vi "Matches.vi"(8 "error in (no error)":errorcluster, 10 "Actual":variant, 11 "Collection Contains in":refnum<class "Collection Contains.lvclass">) -> (0 "error out":errorcluster, 2 "Result":bool, 3 "Collection Contains out":refnum<class "Collection Contains.lvclass">)   [LabVIEW 2017, in "Transparent Assertions.lvlib" / "Collection Contains.lvclass"]
doc: "Evaluates the constraint for <B>Actual</B>. Returns true if the constraint is met."
uses:
  Collection Contains.lvclass
  Collection Contains.lvclass/Collection Contains.ctl
  Transparent Assertions.lvlib
  <vilib>/Utility/Data Type/NI_Data Type.lvlib
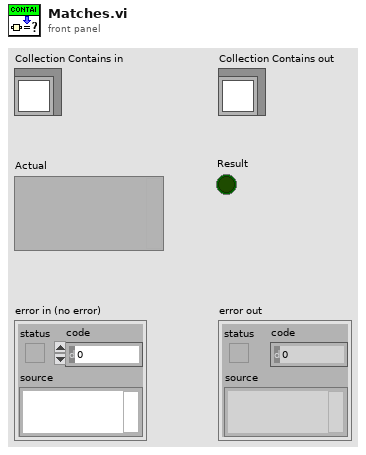
[diagram p1: front panel]
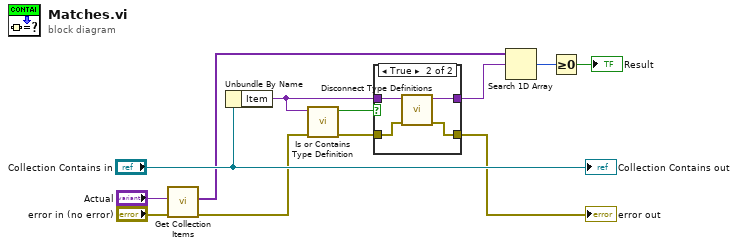
[diagram p0: block diagram]
diagram:
  n1 = call "Get Collection Items.vi"("error in (no error)"="error in (no error)", "Collection"="Actual") -> ("error out"=w3:errorcluster, "Items"=w8:variant[])  [unwired: 8 in]
  n2 = Unbundle By Name("Collection Contains in") -> ("Item"=w4:variant)
  n3 = call <vilib>:"Is or Contains Type Definition.vi"("error in (no error)"=w3, "Variant"=w4) -> ("error out"=w2:errorcluster, "Is or Contains Typedef"=w1:bool)  [unwired: 8 in]
  n4 = case shown="True" w1 {
    tunnel: [w13 w18] -> w6
    tunnel: [w14 w17] -> w5
    tunnel: w4 -> [w13 w16]
    tunnel: w2 -> [w14 w15]
    frame False {
    }
    frame True {
      n5 = call <vilib>:"Disconnect Type Definitions.vi"("error in (no error)"=w15, "Variant in"=w16) -> ("error out"=w17:errorcluster, "Variant out"=w18:variant)  [unwired: 8 in]
    }
  }
  "error out" <- w5
  n6 = Search 1D Array(1D array=w8, element=w6) -> (index of element=w11:i32)  [unwired: 1 in]
  n7 = Greater Or Equal To 0?(x=w11) -> (x >= 0?=→"Result":bool)
  "Collection Contains out" <- "Collection Contains in"
